vi "mastertest.vi"() -> ()   [LabVIEW 2013]
uses:
  dynamic profibus/full response.ctl
  dynamic profibus/profibus master transmit header.ctl
  dynamic profibus/full command.ctl
  dynamic profibus/profibus master action.ctl
  dynamic profibus/parse response value.vi
  <vilib>/FPGAPlugInAG/cRIO-9074/niLvFpga_Open_cRIO-9074.vi
  <vilib>/rvi/interface/common/dynamic/niFpgaDynamicAddResources.vi
  <vilib>/FPGAPlugInAG/Dynamic/niLvFpga_Reset_Dynamic.vi
  <vilib>/FPGAPlugInAG/Dynamic/niLvFpga_Run_Dynamic.vi
  dynamic profibus/read raw commands.vi
  <vilib>/FPGAPlugInAG/Dynamic/niLvFpga_Close_Dynamic.vi
  <vilib>/rvi/interface/nirviOpenFPGA/nirviOpenFPGA.xnode
  FPGA Bitfiles/ProfibusModule_FPGA9074_FPGAMain_bIHCZjrjays.lvbitx
  execution/FPGA Main.vi
  <vilib>/rvi/interface/nirviMethod/nirviMethod.xnode
  <vilib>/rvi/interface/nirviCloseFPGA/nirviCloseFPGA.xnode
  dynamic profibus/dynamic profibus.lvlib
panel:
  in  "send":bool
  in  "milliseconds to wait":u32=1000
  in  "stop":bool
  in  "commands":T1[](array[typedef])=[{"action"=enum."read many inputs", "device"=2, "index"=1, "data"=2}, {"action"=enum."set output", "device"=2, "index"=2, "data"=0}, {"action"=enum."transfer data", "device"=2, "index"=3, "data"=0}, {"action"=enum."transfer diagnostics", "device"=2, "index"=7, "data"=0}, {"action"=enum."get diagnostic", "device"=2, "index"=10, "data"=0}]
  out "responses":T3[](array[typedef])=[{"header"=enum."many inputs", "device"=2, "index"=1, "data"=0}, {"header"=enum."many inputs", "device"=2, "index"=2, "data"=0}, {"header"=enum."Error", "device"=2, "index"=10, "data"=1}]
  out "Slave Info List":T5(array[cluster])=[{"Address"=2, "Input Length"=240, "Output Length"=240}]
  out "error out":errorcluster
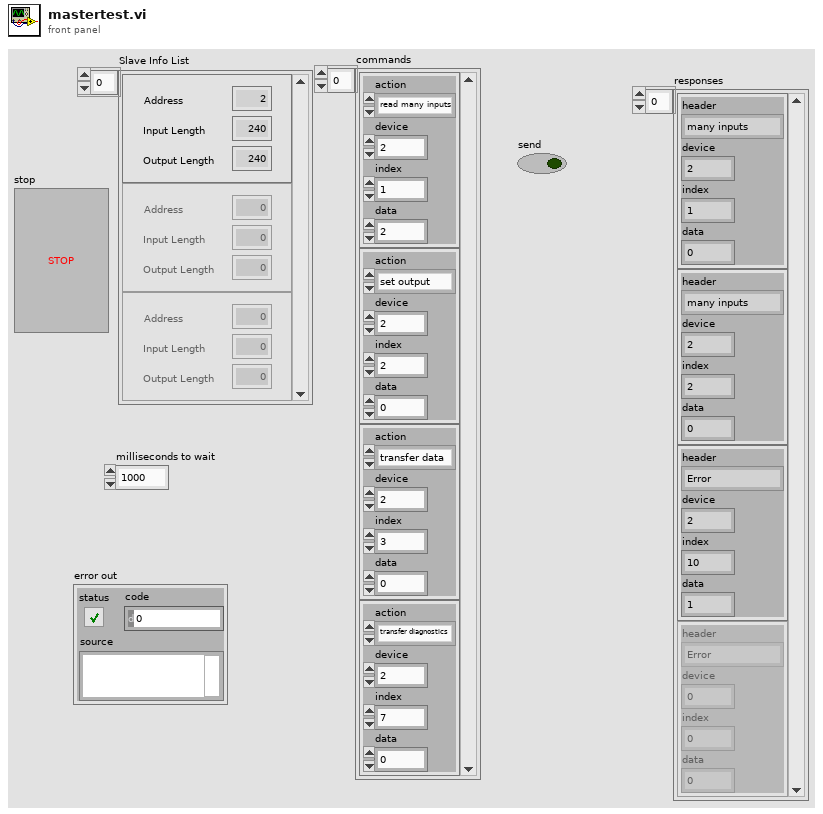
[diagram p1: front panel]
types:
  T1 = typedef "dynamic profibus.lvlib/full command.ctl" = cluster{"action":T2, "device":u8, "index":u8, "data":u8}
  T2 = typedef "dynamic profibus.lvlib/profibus master action.ctl" = enum8{"initialize", "uninitialize", "stop", "get input", "get input size", "set output", "get output size", "get diagnostic", "transfer data", "transfer diagnostics", "read many inputs"}
  T3 = typedef "dynamic profibus.lvlib/full response.ctl" = cluster{"header":T4, "device":u8, "index":u8, "data":u8}
  T4 = typedef "dynamic profibus.lvlib/profibus master transmit header.ctl" = enum8{"Error", "Input", "Diagnostic", "input size", "output size", "many inputs"}
  T5 = cluster{"Address":i8, "Input Length":u8, "Output Length":u8}[]
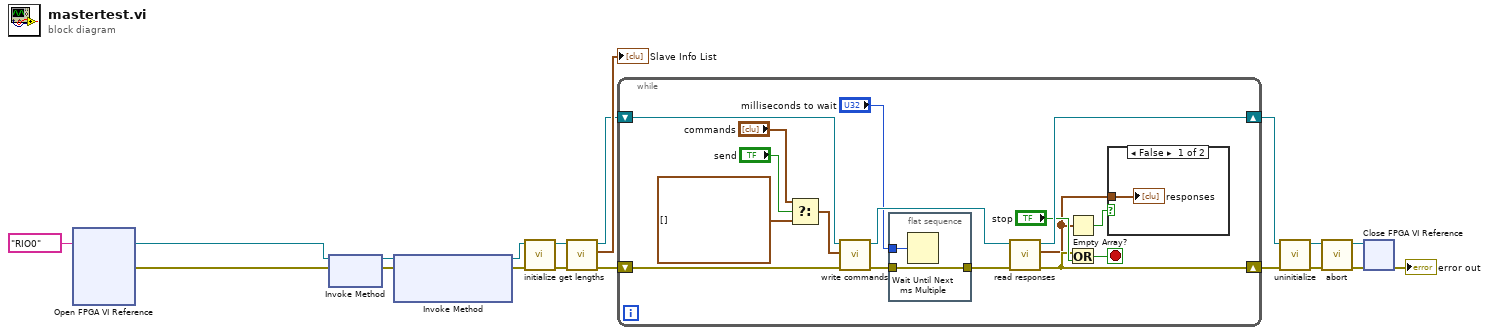
[diagram p0: block diagram]
diagram:
  n1 = xnode "Open FPGA VI Reference"("resource name"=tag "RIO0") -> ("FPGA VI Reference Out"=w15:refnum<k20>, "error out"=w17:errorcluster)  [unwired: 1 in]
  n2 = xnode "Invoke Method"("FPGA VI Reference In"=w15, "error in"=w17) -> ("FPGA VI Reference Out"=w13:refnum<k20>, "error out"=w16:errorcluster)
  n3 = xnode "Invoke Method"("FPGA VI Reference In"=w13, "error in"=w16) -> ("FPGA VI Reference Out"=w12:refnum<k20>, "error out"=w14:errorcluster)  [unwired: 1 in]
  n4 = call "initialize.vi"("error in"=w14, "profibus reference"=w12) -> ("error out"=w19:errorcluster, "profibus reference out"=w18:refnum<k20>)  [unwired: 8 in]
  n5 = call "get lengths.vi"("error in"=w19, "profibus reference"=w18) -> ("error out"=w4:errorcluster, "Slave Info List"=→"Slave Info List":T5, "profibus reference out"=w5:refnum<k20>)  [unwired: 7 in]
  n6 = while {
    shift-right: [w33] -> w3
    shift-left: w5 -> [w35]
    shift-right: [w25] -> w2
    shift-left: w4 -> [w34]
    stop <- w26 stop-if-true
    n7 = Select(t="commands", s="send", f=T1[] []) -> (s? t:f=w30:T1[])
    n8 = call "write commands.vi"("error in"=w34, "commands"=w30, "profibus reference"=w35) -> ("error out"=w23:errorcluster, "profibus reference out"=w32:refnum<k20>)  [unwired: 6 in, 1 out]
    n9 = flat-sequence {
      tunnel: "milliseconds to wait" -> [w38]
      tunnel: [w37] -> w22
      tunnel: w23 -> [w37]
      frame #0 {
        n10 = Wait Until Next ms Multiple(millisecond multiple=w38) -> ()  [unwired: 1 out]
      }
    }
    n11 = call "read responses.vi"("error in"=w22, "profibus reference"=w32) -> ("error out"=w25:errorcluster, "responses"=w20:T3[], "profibus reference out"=w33:refnum<k20>)  [unwired: 7 in]
    n12 = Empty Array?(array=w20) -> (empty?=w21:bool)
    n13 = Or(x=w25, y="stop") -> (x .or. y?=w26:bool)
    n14 = case shown="False" w21 {
      tunnel: w20 -> [w36 _]
      frame False {
        "responses" <- w36
      }
      frame True {
      }
    }
  }
  n15 = call "uninitialize.vi"("error in"=w2, "profibus reference"=w3) -> ("error out"=w10:errorcluster, "profibus reference out"=w11:refnum<k20>)  [unwired: 8 in]
  n16 = call "abort.vi"("error in"=w10, "profibus reference"=w11) -> ("error out"=w8:errorcluster, "profibus reference out"=w9:refnum<k20>)  [unwired: 8 in]
  n17 = xnode "Close FPGA VI Reference"("FPGA VI Reference In"=w9, "error in"=w8) -> ("error out"=→"error out":errorcluster)
